vi "Button and Switch CCS.vi"() -> ()   [LabVIEW 2021]
uses:
  <vilib>/addons/control/pid/autopid.llb/PID autotuning parameters (adv).ctl
  <vilib>/Instr/_visa.llb/VISA Configure Serial Port (Instr).vi
  <vilib>/addons/control/pid/NI_PID_autopid.lvlib
  <vilib>/ptbypt/NI_PtbyPt.lvlib
panel:
  in  "ACCEPT ACC PID":bool
  in  "auto? (F) 2":bool
  out "tuned PID gains 2":T1={"proportional gain (Kc)"=1.0, "integral time (Ti, min)"=0.01, "derivative time (Td, min)"=0.0} {"derivative time (Td, min)" format="%#.6g"; "integral time (Ti, min)" format="%#.6g"; "proportional gain (Kc)" format="%#.6g"}
  out "tuning completed?":bool
  in  "autotuning parameters 2":T2={"technique"=2, "type of controller"=1, "control specification"=0, "amplitude"=1.0} {"amplitude" format="%.2f"; "control specification" items=["normal", "fast", "slow"]; "type of controller" items=["P", "PI", "PID"]; "technique" items=["Step Open Loop", "Step Closed Loop", "Relay", "PID Relay"]}
  in  "reinitialize? (F) 2":bool
  in  "PID gains 2":T1={"proportional gain (Kc)"=1.0, "integral time (Ti, min)"=0.01, "derivative time (Td, min)"=0.0} {"derivative time (Td, min)" format="%#.6g"; "integral time (Ti, min)" format="%#.6g"; "proportional gain (Kc)" format="%#.6g"}
  in  "autotune? (F) 2":bool
  out "Target Distance (m)":dbl
  out "Time Level":dbl=125.0
  out "Distance (m)":i8=4
  out "Brake Light":bool
  in  "VISA resource name":refnum<visa-resource-name>="COM3"
  in  "baud rate":u32=115200
  out "RPM":i64(knob) scale=0.0..650.0
  out "VELOCITY":u64(knob) scale=0.0..200.0
  out "GAS PEDAL":u8(slide) scale=0.0..255.0
  out "BRAKE PEDAL":u8(slide)=1 scale=0.0..255.0
  out "VELOCITY":cluster{"VELOCITY":u64, "Cruise Setpoint":u64}(graph)
  in  "autotune? (F)":bool
  in  "PID gains":T1={"proportional gain (Kc)"=0.453862, "integral time (Ti, min)"=0.006883, "derivative time (Td, min)"=0.0} {"derivative time (Td, min)" format="%#.6g"; "integral time (Ti, min)" format="%#.6g"; "proportional gain (Kc)" format="%#.6g"}
  in  "dt (s)":dbl=0.021
  in  "reinitialize? (F)":bool
  in  "autotuning parameters":T2={"technique"=0, "type of controller"=1, "control specification"=1, "amplitude"=30.0} {"amplitude" format="%.2f"; "control specification" items=["normal", "fast", "slow"]; "type of controller" items=["P", "PI", "PID"]; "technique" items=["Step Open Loop", "Step Closed Loop", "Relay", "PID Relay"]}
  out "completed?":bool
  out "tuned PID gains":T1={"proportional gain (Kc)"=0.453862, "integral time (Ti, min)"=0.006883, "derivative time (Td, min)"=0.0} {"derivative time (Td, min)" format="%#.6g"; "integral time (Ti, min)" format="%#.6g"; "proportional gain (Kc)" format="%#.6g"}
  in  "auto? (F)":bool
  in  "ACCEPT SPEED PID":bool
  out "MOTOR CONTROL":dbl(graph)
  in  "stop":bool
  in  "PID Mode":i64(knob)=2 scale=1.0..3.0
  in  "Cruise Enable":bool
  in  "Distance":bool
  out "Distance Level":i8=4
  out "Cruise Active":bool
  out "Cruise Setpoint":u64=125
  in  "Speed +":bool
  in  "Speed -":bool
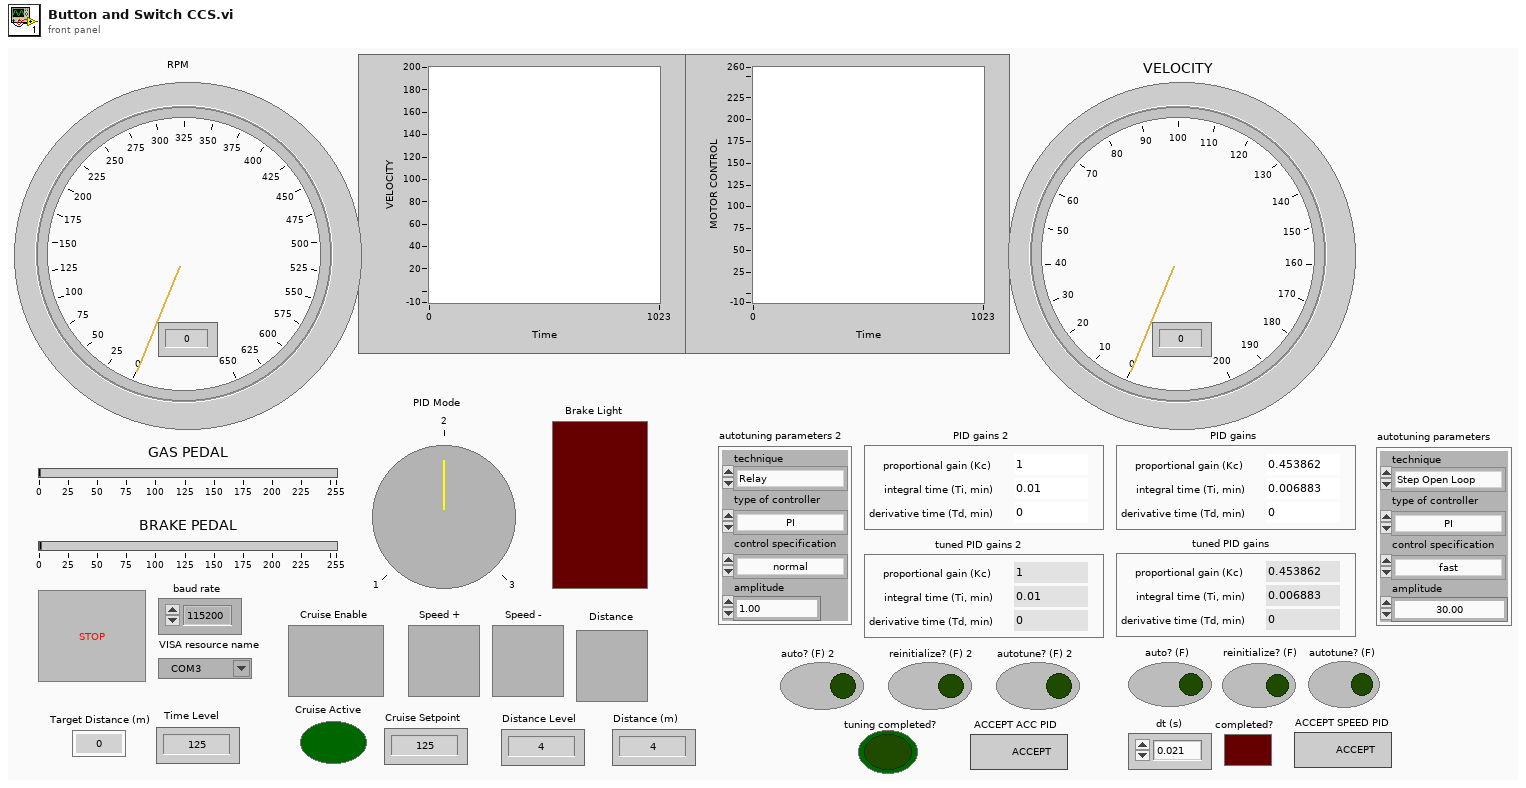
[diagram p1: front panel]
types:
  T1 = cluster{"proportional gain (Kc)":dbl, "integral time (Ti, min)":dbl, "derivative time (Td, min)":dbl}
  T2 = typedef "NI_PID_autopid.lvlib/PID autotuning parameters (adv).ctl" = cluster{"technique":u16, "type of controller":u16, "control specification":u16, "amplitude":dbl}
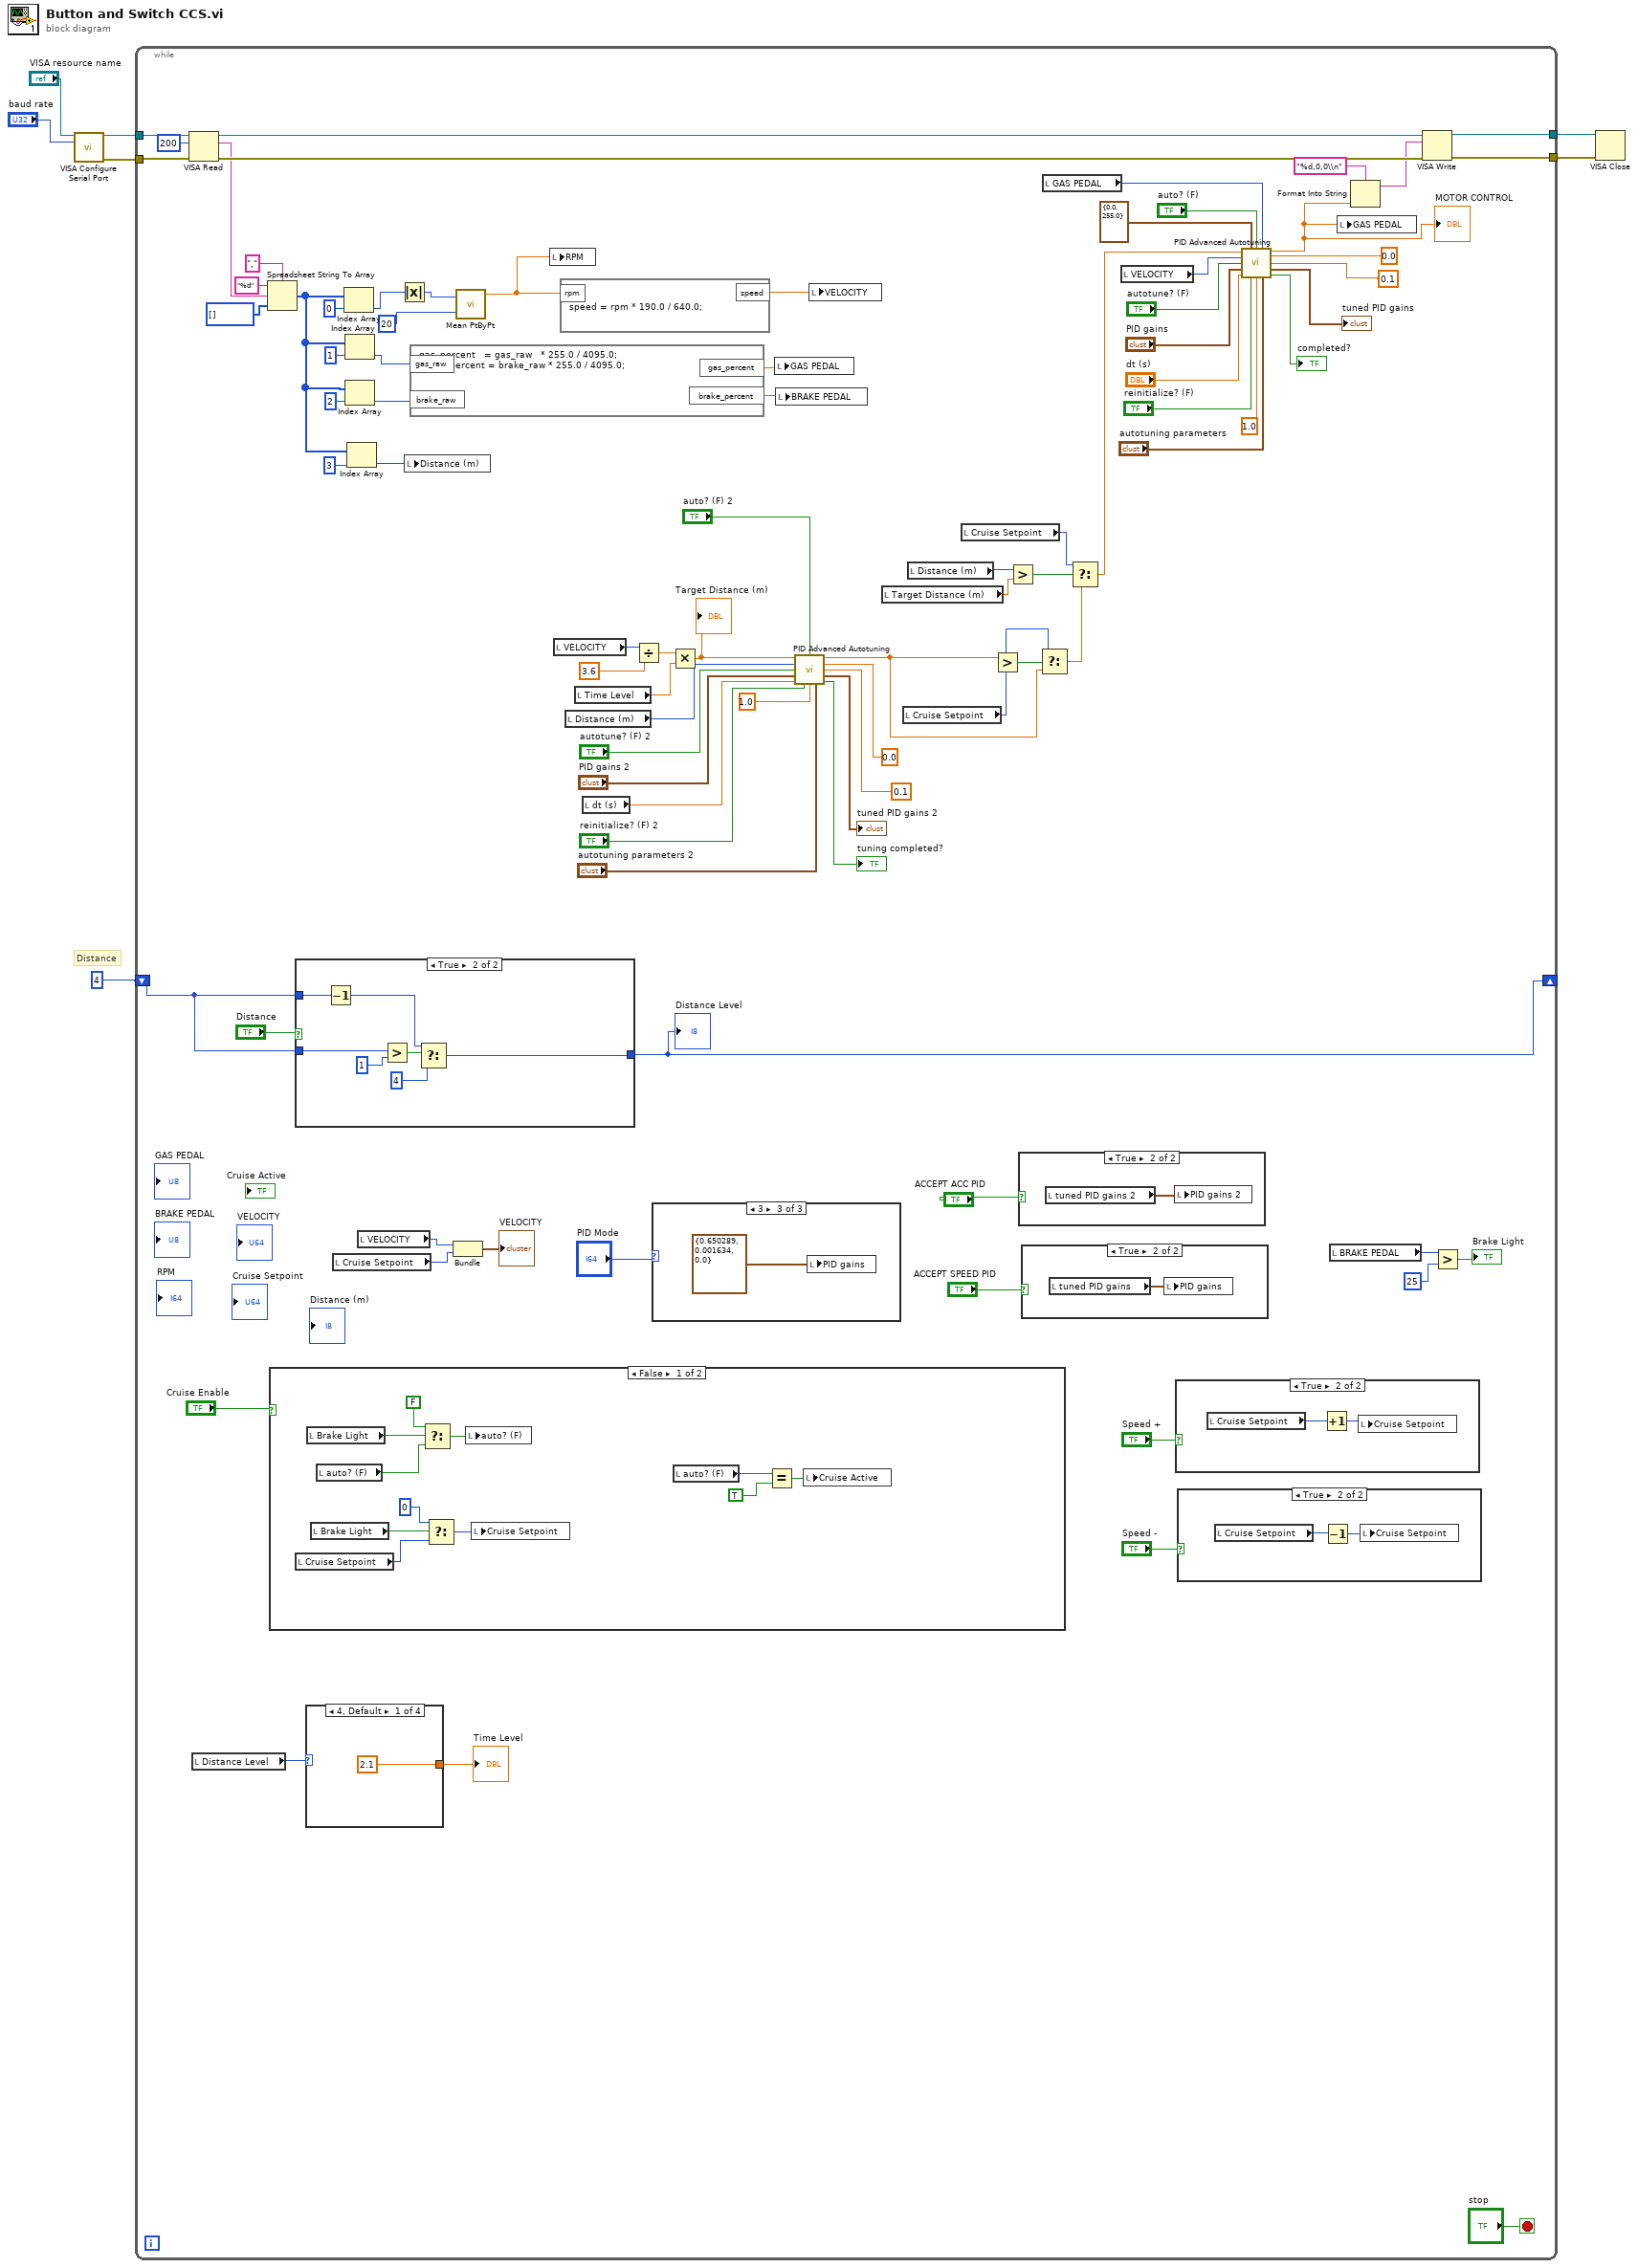
[diagram p0: block diagram]
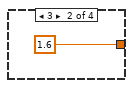
[diagram p3: hidden frame]
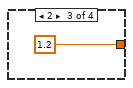
[diagram p4: hidden frame]
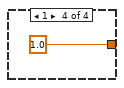
[diagram p5: hidden frame]
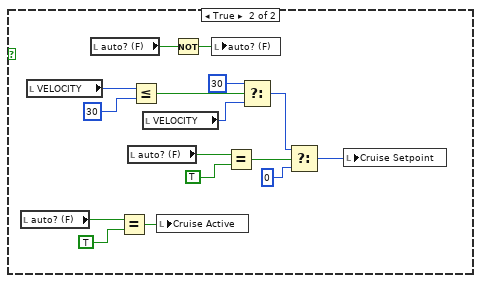
[diagram p9: hidden frame]
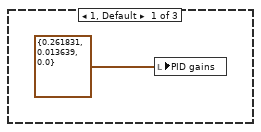
[diagram p10: hidden frame]
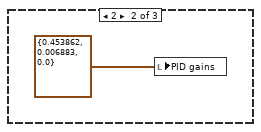
[diagram p11: hidden frame]
diagram:
  # "Distance"
  n1 = call-poly "VISA Configure Serial Port"("VISA resource name"="VISA resource name", "baud rate (9600)"="baud rate") -> ("VISA resource name out"=w6:refnum<visa-resource-name>, "error out"=w5:errorcluster)  [unwired: 12 in]
  n2 = while {
    tunnel: w6 -> [w94]
    tunnel: w5 -> [w93]
    tunnel: [w68] -> w4
    tunnel: [w69] -> w3
    shift-right: [w43] -> _
    shift-left: i64 4 ("f") -> [w44]
    stop <- "stop" stop-if-true
    n3 = VISA Read(VISA resource name=w94, byte count=u32 200, error in (no error)=w93) -> (VISA resource name out=w91:refnum<visa-resource-name>, read buffer=w89:string, error out=w92:errorcluster)  [unwired: 1 out]
    n4 = local read "Distance Level"() -> (w36:i8)
    n5 = Spreadsheet String To Array(delimiter (Tab)=",", format string="%d", spreadsheet string=w89, array type (2D Dbl)=i32[] []) -> (array=w39:i32[])
    n6 = case shown="False" "Cruise Enable" {
      frame False {
        n7 = local read "Cruise Setpoint"() -> (w114:u64)
        n8 = local read "Brake Light"() -> (w122:bool)
        n9 = local read "Brake Light"() -> (w115:bool)
        n10 = local read "auto? (F)"() -> (w119:bool)
        n11 = Select(t=FALSE, s=w122, f=w119) -> (s? t:f=w120:bool)
        n12 = Select(t=u64 0, s=w115, f=w114) -> (s? t:f=w112:u64)
        n13 = local write "auto? (F)"(w120) -> ()
        n14 = local write "Cruise Setpoint"(w112) -> ()
        n15 = local read "auto? (F)"() -> (w117:bool)
        n16 = Equal?(x=w117, y=TRUE) -> (x = y?=w116:bool)
        n17 = local write "Cruise Active"(w116) -> ()
      }
      frame True {
        n18 = local read "auto? (F)"() -> (w130:bool)
        n19 = local read "VELOCITY"() -> (w129:u64)
        n20 = local read "auto? (F)"() -> (w138:bool)
        n21 = Equal?(x=w130, y=TRUE) -> (x = y?=w123:bool)
        n22 = local read "auto? (F)"() -> (w136:bool)
        n23 = Less Or Equal?(x=w129, y=u64 30) -> (x <= y?=w127:bool)
        n24 = local read "VELOCITY"() -> (w126:u64)
        n25 = local write "Cruise Active"(w123) -> ()
        n26 = Not(x=w138) -> (.not. x?=w137:bool)
        n27 = local write "auto? (F)"(w137) -> ()
        n28 = Equal?(x=w136, y=TRUE) -> (x = y?=w134:bool)
        n29 = Select(t=u64 30, s=w127, f=w126) -> (s? t:f=w124:u64)
        n30 = Select(t=w124, s=w134, f=i64 0) -> (s? t:f=w133:u64)
        n31 = local write "Cruise Setpoint"(w133) -> ()
      }
    }
    n32 = case shown="True" "Distance" {
      tunnel: w44 -> [w100 w107]
      tunnel: w44 -> [_ w106]
      tunnel: [w100 w101] -> w43
      frame False {
      }
      frame True {
        n33 = Decrement(x=w107) -> (x-1=w103:i64)
        n34 = Greater?(x=w106, y=i64 1) -> (0:w104:bool)
        n35 = Select(t=w103, s=w104, f=i64 4) -> (s? t:f=w101:i64)
      }
    }
    "Distance Level" <- w43
    n36 = case shown="4, Default" w36 {
      tunnel: [2.1 ("Time Level") 1.6 ("Time Level") 1.2 ("Time Level") 1.0 ("Time Level")] -> w35
      frame 4, Default {
      }
      frame 3 {
      }
      frame 2 {
      }
      frame 1 {
      }
    }
    "Time Level" <- w35
    n37 = local read "Cruise Setpoint"() -> (w48:u64)
    n38 = Index Array(array=w39, index=0) -> (element=w61:i32)
    n39 = Index Array(array=w39, index=1) -> (element=w65:i32)
    n40 = Index Array(array=w39, index=2) -> (element=w64:i32)
    n41 = Index Array(array=w39, index=3) -> (element=w37:i32)
    n42 = local read "VELOCITY"() -> (w56:u64)
    n43 = Absolute Value(x=w61) -> (abs(x)=w60:i32)
    n44 = local write "Distance (m)"(w37) -> ()
    n45 = formula code="gas_percent   = gas_raw   * 255.0 / 4095.0;\nbrake_percent = brake_raw * 255.0 / 4095.0;"("gas_raw"=w65, "brake_raw"=w64) -> ("gas_percent"=w63:dbl, "brake_percent"=w62:dbl)
    n46 = Bundle("VELOCITY"=w56, "Cruise Setpoint"=w48) -> (→"VELOCITY":cluster{"VELOCITY":u64, "Cruise Setpoint":u64})  [unwired: 1 in]
    n47 = call <vilib>:"Mean PtByPt.vi"("x"=w60, "sample length"=20) -> ("mean"=w66:dbl)  [unwired: 2 in, 1 out]
    n48 = local write "RPM"(w66) -> ()
    n49 = local read "VELOCITY"() -> (w33:u64)
    n50 = formula code="speed = rpm * 190.0 / 640.0;"("rpm"=w66) -> ("speed"=w67:dbl)
    n51 = local read "Distance (m)"() -> (w24:i8)
    n52 = local read "Time Level"() -> (w31:dbl)
    n53 = local read "dt (s)"() -> (w21:dbl)
    n54 = Divide(x=w33, y=3.6) -> (x/y=w32:dbl)
    n55 = case shown="3" "PID Mode" {
      frame 1, Default {
        n56 = local write "PID gains"(T1 {"proportional gain (Kc)"=0.261831, "integral time (Ti, min)"=0.013639, "derivative time (Td, min)"=0.0} ("PID gains")) -> ()
      }
      frame 2 {
        n57 = local write "PID gains"(T1 {"proportional gain (Kc)"=0.453862, "integral time (Ti, min)"=0.006883, "derivative time (Td, min)"=0.0} ("PID gains")) -> ()
      }
      frame 3 {
        n58 = local write "PID gains"(T1 {"proportional gain (Kc)"=0.650289, "integral time (Ti, min)"=0.001634, "derivative time (Td, min)"=0.0} ("PID gains")) -> ()
      }
    }
    n59 = Multiply(x=w32, y=w31) -> (x*y=w25:dbl)
    "Target Distance (m)" <- w25
    n60 = local write "GAS PEDAL"(w63) -> ()
    n61 = local write "BRAKE PEDAL"(w62) -> ()
    n62 = call <vilib>:"PID Advanced Autotuning.vi"("setpoint"=w25, "auto? (F)"="auto? (F) 2", "process variable"=w24, "gamma"=0.0, "autotune? (F)"="autotune? (F) 2", "alpha"=0.1, "PID gains"="PID gains 2", "dt (s)"=w21, "reinitialize? (F)"="reinitialize? (F) 2", "beta"=1.0, "autotuning parameters"="autotuning parameters 2") -> ("output"=w10:dbl, "tuned PID gains"=→"tuned PID gains 2":T1, "tuning completed?"=→"tuning completed?":bool)  [unwired: 2 in]
    n63 = local write "VELOCITY"(w67) -> ()
    n64 = local read "Target Distance (m)"() -> (w29:dbl)
    n65 = local read "Cruise Setpoint"() -> (w9:u64)
    n66 = local read "Distance (m)"() -> (w30:i8)
    n67 = local read "Cruise Setpoint"() -> (w27:u64)
    n68 = Greater?(x=w10, y=w9) -> (0:w12:bool)
    n69 = Greater?(x=w30, y=w29) -> (0:w28:bool)
    n70 = case shown="True" "ACCEPT ACC PID" {
      frame False {
      }
      frame True {
        n71 = local read "tuned PID gains 2"() -> (w95:T1)
        n72 = local write "PID gains 2"(w95) -> ()
      }
    }
    n73 = case shown="True" "ACCEPT SPEED PID" {
      frame False {
      }
      frame True {
        n74 = local read "tuned PID gains"() -> (w142:T1)
        n75 = local write "PID gains"(w142) -> ()
      }
    }
    n76 = Select(t=w9, s=w12, f=w10) -> (s? t:f=w11:dbl)
    n77 = local read "GAS PEDAL"() -> (w51:u8)
    n78 = Select(t=w27, s=w28, f=w11) -> (s? t:f=w26:dbl)
    n79 = local read "VELOCITY"() -> (w80:u64)
    n80 = case shown="True" "Speed +" {
      frame False {
      }
      frame True {
        n81 = local read "Cruise Setpoint"() -> (w110:u64)
        n82 = Increment(x=w110) -> (x+1=w111:u64)
        n83 = local write "Cruise Setpoint"(w111) -> ()
      }
    }
    n84 = case shown="True" "Speed -" {
      frame False {
      }
      frame True {
        n85 = local read "Cruise Setpoint"() -> (w109:u64)
        n86 = Decrement(x=w109) -> (x-1=w108:u64)
        n87 = local write "Cruise Setpoint"(w108) -> ()
      }
    }
    n88 = call <vilib>:"PID Advanced Autotuning.vi"("setpoint"=w26, "output range"=cluster{"output high":dbl, "output low":dbl} {"output high"=0.0, "output low"=255.0}, "auto? (F)"="auto? (F)", "manual control"=w51, "process variable"=w80, "gamma"=0.0, "autotune? (F)"="autotune? (F)", "alpha"=0.1, "PID gains"="PID gains", "dt (s)"="dt (s)", "reinitialize? (F)"="reinitialize? (F)", "beta"=1.0, "autotuning parameters"="autotuning parameters") -> ("output"=w50:dbl, "tuned PID gains"=→"tuned PID gains":T1, "tuning completed?"=→"completed?":bool)
    "MOTOR CONTROL" <- w50
    n89 = local read "BRAKE PEDAL"() -> (w42:u8)
    n90 = local write "GAS PEDAL"(w50) -> ()
    n91 = Format Into String(format string="%d,0,0\\n", w50) -> (resulting string=w81:string)  [unwired: 2 in, 1 out]
    n92 = VISA Write(VISA resource name=w91, write buffer=w81, error in (no error)=w92) -> (VISA resource name out=w69:refnum<visa-resource-name>, error out=w68:errorcluster)  [unwired: 1 out]
    n93 = Greater?(x=w42, y=u8 25) -> (0:→"Brake Light":bool)
  }
  n94 = VISA Close(VISA resource name=w3, error in (no error)=w4) -> ()  [unwired: 1 out]
